vi "Save_Points(X-Y)_Areas-1.vi"(3 "error IN":errorcluster, 5 "[IN] Cluster of \npoints and areas":T1(array[cluster])) -> (0 "error OUT":errorcluster, 1 "[OUT] Areas":dbl[][](array[numeric]), 2 "[OUT] Points (X,Y)":dbl[][](array[numeric]))   [LabVIEW 2013]
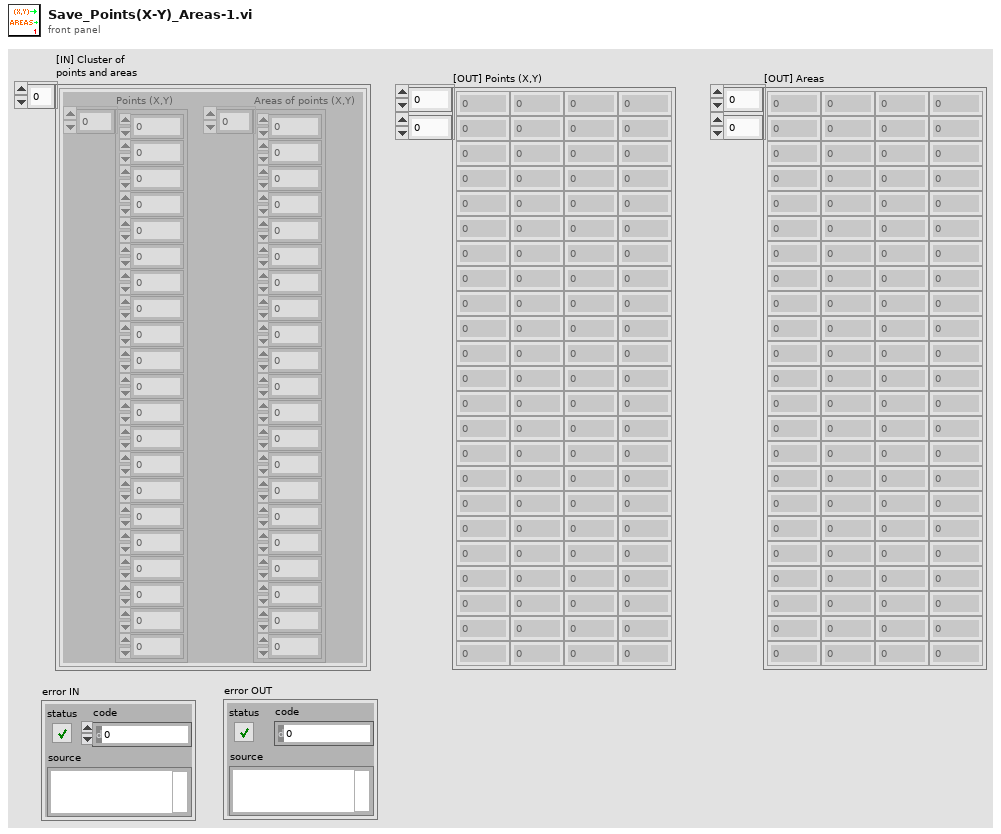
[diagram p1: front panel]
types:
  T1 = cluster{"Points (X,Y)":dbl[], "Areas of points (X,Y)":dbl[]}[]
  T2 = cluster{"Points (X,Y)":dbl[], "Areas of points (X,Y)":dbl[]}
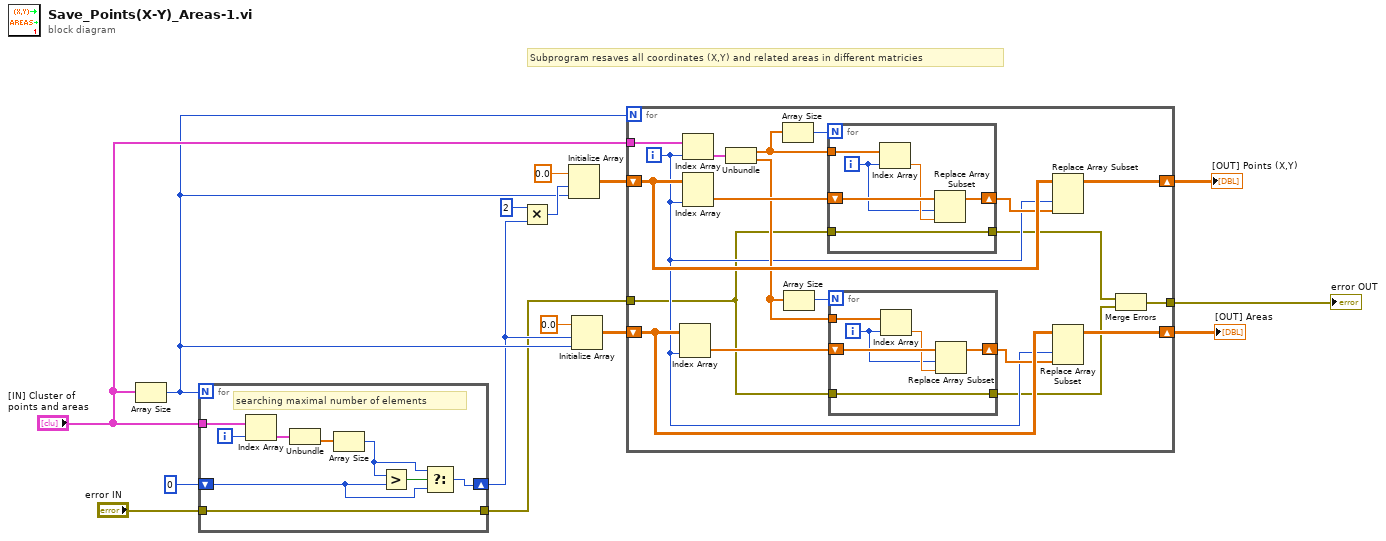
[diagram p0: block diagram]
diagram:
  # "Subprogram resaves all coordinates (X,Y) and related areas in different matricies"
  n1 = Array Size(array="[IN] Cluster of \npoints and areas") -> (size(s)=w7:i32)
  n2 = for {
    N: w7 -> [_]
    tunnel: "[IN] Cluster of \npoints and areas" -> [w24]
    shift-right: [w19] -> w5
    shift-left: 0 -> [w16]
    tunnel: "error IN" -> [w18]
    tunnel: [w18] -> w4
    i -> [w23]
    # "searching maximal number of elements"
    n3 = Index Array(array=w24, index=w23) -> (element=w22:T2)
    n4 = Unbundle(w22) -> ("Areas of points (X,Y)"=w21:dbl[])  [unwired: 1 out]
    n5 = Array Size(array=w21) -> (size(s)=w17:i32)
    n6 = Greater?(x=w17, y=w16) -> (0:w20:bool)
    n7 = Select(t=w17, s=w20, f=w16) -> (s? t:f=w19:i32)
  }
  n8 = Multiply(x=2, y=w5) -> (x*y=w11:i32)
  n9 = Initialize Array(0.0 ("element"), w11, w7) -> (w9:dbl[][])
  n10 = Initialize Array(0.0 ("element"), w5, w7) -> (w6:dbl[][])
  n11 = for {
    N: w7 -> [_]
    tunnel: "[IN] Cluster of \npoints and areas" -> [w43]
    shift-right: [w36] -> w2
    shift-left: w9 -> [w38]
    shift-right: [w31] -> w1
    shift-left: w6 -> [w32]
    tunnel: w4 -> [w28]
    tunnel: [w25] -> w3
    i -> [w29]
    n12 = Index Array(array=w32, index (col)=w29) -> (element=w33:dbl[])  [unwired: 1 in]
    n13 = Index Array(array=w43, index=w29) -> (element=w42:T2)
    n14 = Index Array(array=w38, index (col)=w29) -> (element=w40:dbl[])  [unwired: 1 in]
    n15 = Unbundle(w42) -> ("Points (X,Y)"=w39:dbl[], "Areas of points (X,Y)"=w34:dbl[])
    n16 = Array Size(array=w39) -> (size(s)=w41:i32)
    n17 = Array Size(array=w34) -> (size(s)=w35:i32)
    n18 = for {
      N: w41 -> [_]
      shift-right: [w51] -> w37
      shift-left: w40 -> [w55]
      tunnel: w39 -> [w54]
      tunnel: w28 -> [w50]
      tunnel: [w50] -> w26
      i -> [w52]
      n19 = Index Array(array=w54, index=w52) -> (element=w53:dbl)
      n20 = Replace Array Subset(array=w55, new element=w53, index=w52) -> (w51:dbl[])
    }
    n21 = for {
      N: w35 -> [_]
      shift-right: [w45] -> w30
      shift-left: w33 -> [w49]
      tunnel: w34 -> [w48]
      tunnel: w28 -> [w44]
      tunnel: [w44] -> w27
      i -> [w46]
      n22 = Index Array(array=w48, index=w46) -> (element=w47:dbl)
      n23 = Replace Array Subset(array=w49, new element=w47, index=w46) -> (w45:dbl[])
    }
    n24 = Replace Array Subset(array=w38, new element=w37, index (col)=w29) -> (w36:dbl[][])  [unwired: 1 in]
    n25 = Replace Array Subset(array=w32, new element=w30, index (col)=w29) -> (w31:dbl[][])  [unwired: 1 in]
    n26 = Merge Errors(w26, w27) -> (w25:errorcluster)
  }
  "error OUT" <- w3
  "[OUT] Points (X,Y)" <- w2
  "[OUT] Areas" <- w1
